vi "HelloWorld.vi"() -> ()   [LabVIEW 2020, in "LibraryExample.lvlib"]
uses:
  LibraryExample.lvlib
panel:
  out "Out":string
  in  "In":string
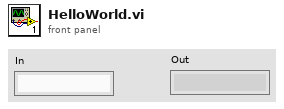
[diagram p1: front panel]
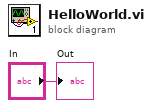
[diagram p0: block diagram]
diagram:
  "Out" <- "In"
